vi "RT Driver VI.vi"(7 "Operation":T1, 11 "Device Reference in":T2 format="%.0x") -> (0 "Error Code":i32)   [LabVIEW 2014, in "Scriptable Model Interface Engine.lvlib"]
uses:
  Scriptable Model Interface Engine.lvlib
  runtime state.ctl
  Shared/model parameters.ctl
  Shared/Scriptable Model Interface Shared.lvlib
  <vilib>/NI Veristand/Custom Device API/Model Interface Driver VI Operation.ctl
  <vilib>/NI Veristand/Custom Device API/Custom Device API.lvlib
  <vilib>/NI Veristand/Custom Device API/Custom Device Item Ref.ctl
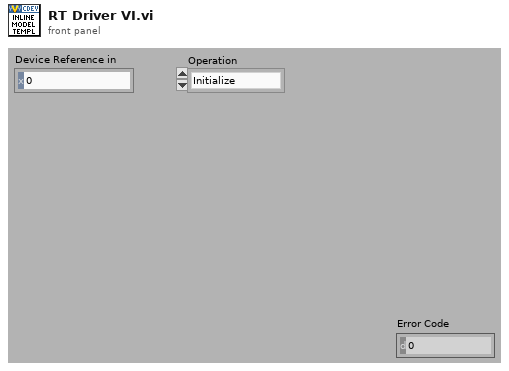
[diagram p1: front panel]
types:
  T1 = typedef "Custom Device API.lvlib/Model Interface Driver VI Operation.ctl" = enum16{"Initialize", "Start", "Execute Model", "Close"}
  T2 = typedef "Custom Device API.lvlib/Custom Device Item Ref.ctl" = u64
  T3 = typedef "Scriptable Model Interface Engine.lvlib/runtime state.ctl" = cluster{"model parameters":T4}
  T4 = typedef "Scriptable Model Interface Shared.lvlib/model parameters.ctl" = cluster{"p":dbl}
  T5 = typedef "Custom Device API.lvlib/Data Reference.ctl" = i32
  T6 = typedef "Scriptable Model Interface Shared.lvlib/model inputs.ctl" = cluster{"i":dbl}
  T7 = typedef "Scriptable Model Interface Shared.lvlib/model outputs.ctl" = cluster{"o":dbl}
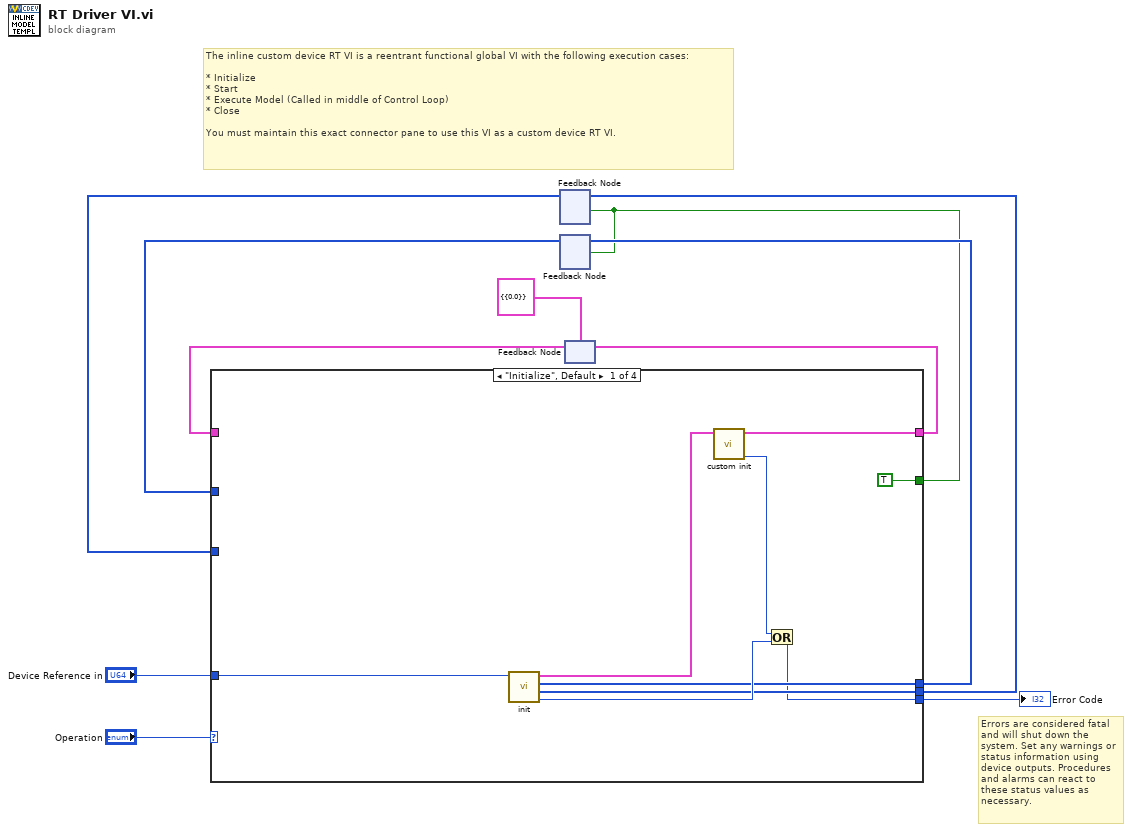
[diagram p0: block diagram]
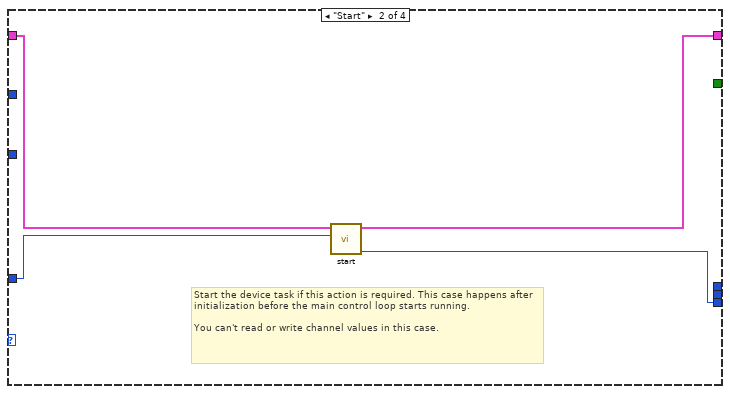
[diagram p2: hidden frame]
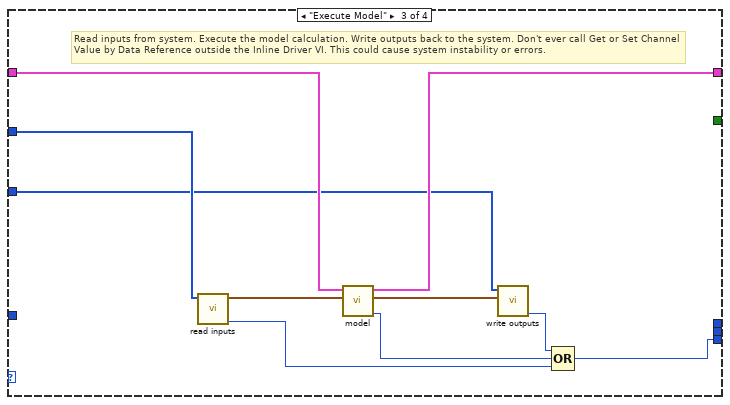
[diagram p3: hidden frame]
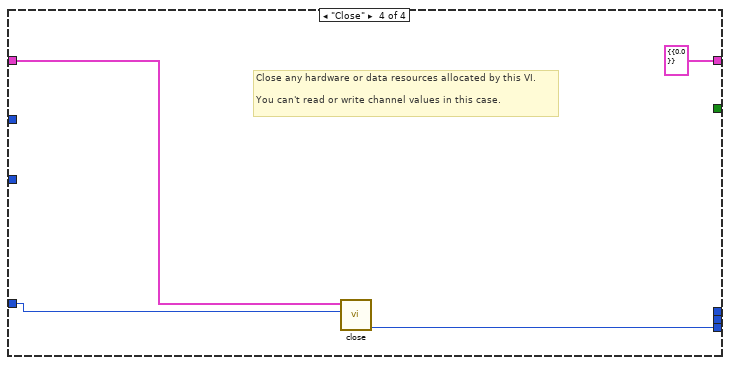
[diagram p4: hidden frame]
diagram:
  # "Errors are considered fatal and will shut down the system. Set any warnings or status information using device outputs. Procedures and alarms can react to these status values as necessary."
  # "The inline custom device RT VI is a reentrant functional global VI with the following execution cases:\n\n* Initialize\n* Start\n* Execute Model (Called in middle of Control Loop)\n* Close\n\nYou must maintain this exact connector pane to use this VI as a custom device RT VI."
  n1 = feedback #1() -> (w2:T5[])  [unwired: 1 out]
  n2 = feedback #2() -> (w3:T5[])  [unwired: 1 out]
  n3 = feedback #3(T3 {"model parameters"={"p"=0.0}} ("cluster")) -> (w9:T3)
  n4 = case shown="\"Initialize\", Default" "Operation" {
    tunnel: [w14 w22 w28 T3 {"model parameters"={"p"=0.0}} ("cluster")] -> w10
    tunnel: w9 -> [_ w23 w29 w37]
    tunnel: "Device Reference in" -> [w20 w21 _ w35]
    tunnel: [w13 w24 w31 w36] -> w7
    tunnel: [w18 _ _ _] -> w5
    tunnel: [w17 _ _ _] -> w4
    tunnel: w3 -> [_ _ w27 _]
    tunnel: w2 -> [_ _ w25 _]
    tunnel: [TRUE _ _ _] -> w1
    frame "Initialize", Default {
      n5 = call "init.vi"("Device Reference in"=w20) -> ("error code"=w19:i32, "outputs"=w17:T5[], "inputs"=w18:T5[], "state"=w15:T3)  [unwired: 7 in]
      n6 = call "custom init.vi"("state"=w15) -> ("abort code"=w12:i32, "state out"=w14:T3)  [unwired: 9 in]
      n7 = Or(x=w12, y=w19) -> (x .or. y?=w13:i32)
    }
    frame "Start" {
      # "Start the device task if this action is required. This case happens after initialization before the main control loop starts running.\n\nYou can't read or write channel values in this case."
      n8 = call "start.vi"("Device Reference in"=w21, "state in"=w23) -> ("code"=w24:i32, "state out"=w22:T3)  [unwired: 8 in]
    }
    frame "Execute Model" {
      # "Read inputs from system. Execute the model calculation. Write outputs back to the system. Don't ever call Get or Set Channel Value by Data Reference outside the Inline Driver VI. This could cause system instability or errors."
      n9 = call "read inputs.vi"("inputs"=w27) -> ("code"=w32:i32, "model inputs"=w26:T6)  [unwired: 9 in]
      n10 = call "model.vi"("model inputs"=w26, "state in"=w29) -> ("abort code"=w33:i32, "model outputs"=w30:T7, "state out"=w28:T3)  [unwired: 7 in]
      n11 = call "write outputs.vi"("model outputs"=w30, "outputs"=w25) -> ("code"=w34:i32)  [unwired: 9 in]
      n12 = Compound Arithmetic op=OR(w34, w33, w32) -> (w31:i32)
    }
    frame "Close" {
      # "Close any hardware or data resources allocated by this VI.\n\nYou can't read or write channel values in this case."
      n13 = call "close.vi"("Device Reference in"=w35, "state"=w37) -> ("code"=w36:i32)  [unwired: 9 in]
    }
  }
  "Error Code" <- w7
  n14 = feedback-in #1(w4, w1) -> ()
  n15 = feedback-in #2(w5, w1) -> ()
  n16 = feedback-in #3(w10) -> ()
